vi "IDS_system_errorNumberToRecommendation.vi"(8 "errorNumber":i32, 9 "language":u32, 10 "deviceHandle":i32) -> (1 "recommendation String":string, 3 "deviceHandle out":i32)   [LabVIEW 2016]
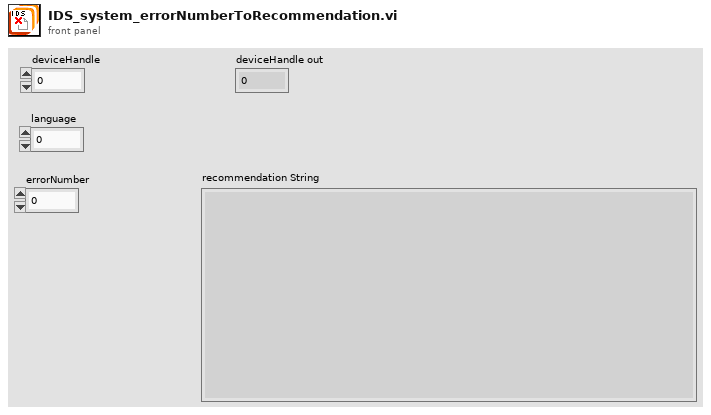
[diagram p1: front panel]
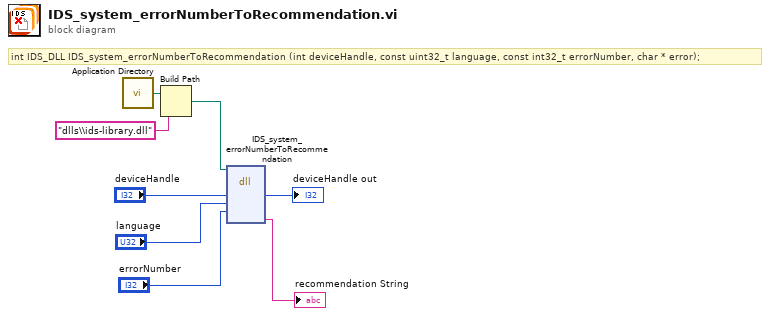
[diagram p0: block diagram]
diagram:
  # "int IDS_DLL IDS_system_errorNumberToRecommendation (int deviceHandle, const uint32_t language, const int32_t errorNumber, char * error);"
  n1 = call <vilib>:"Application Directory.vi"() -> ("Application Directory"=w3:path)
  n2 = Build Path(base path=w3, name or relative path="dlls\\ids-library.dll" ("ipAddress")) -> (appended path=w1:path)
  n3 = dll-call lib="C:/Users/matheus/Desktop/LabVIEW_Draft_V1.6.0/dlls/ids-library.dll" fn="IDS_system_errorNumberToRecommendation"(path in=w1, "deviceHandle"="deviceHandle", "language"="language", "errorNumber"="errorNumber") -> ("deviceHandle"=→"deviceHandle out":i32, "recommendation"=→"recommendation String":string)  [unwired: 6 in, 2 out]
